vi "Read Function Definition.vi"(8 "error in":errorcluster, 11 "Modbus master in":refnum<class "Modbus Master.lvclass">) -> (0 "error out":errorcluster, 2 "master function definition":refnum<class "Master Function Definition.lvclass">, 3 "Modbus master out":refnum<class "Modbus Master.lvclass">)   [LabVIEW 2015, in "Modbus Library.lvlib" / "Modbus Master.lvclass"]
doc: "This VI is an accessor for the function definition stored in the Modbus master instance. This accessor can be used as a property node. This function definition is used by the master to determine how to pack and unpack Modbus protocol data units."
uses:
  Modbus Master.lvclass
  Master Function Definition/Master Function Definition.lvclass
  Modbus Master.lvclass/Modbus Master.ctl
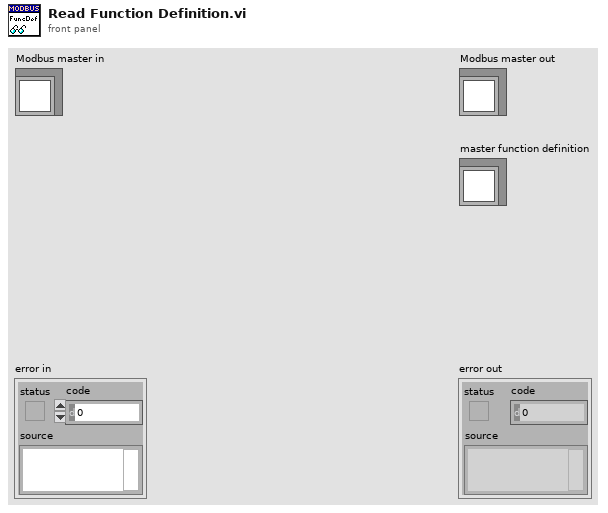
[diagram p1: front panel]
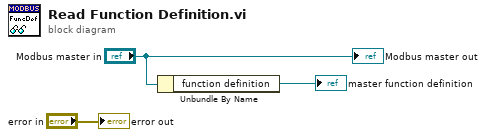
[diagram p0: block diagram]
diagram:
  n1 = Unbundle By Name("Modbus master in") -> ("function definition"=→"master function definition":refnum<class "Master Function Definition.lvclass">)
  "error out" <- "error in"
  "Modbus master out" <- "Modbus master in"
